vi "type_A_uncertainty.vi"(11 "X":dbl[](array[numeric]) format="%0.2f") -> (1 "u_A(x)":dbl, 3 "mean":dbl format="%0.2f")   [LabVIEW 2021]
uses:
  <vilib>/Analysis/NI_AALBase.lvlib
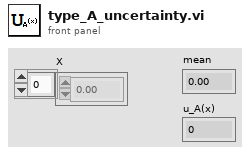
[diagram p1: front panel]
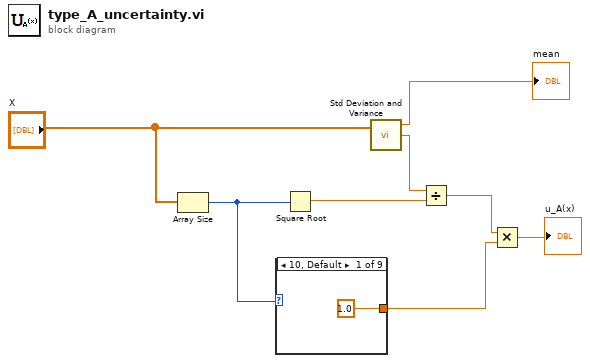
[diagram p0: block diagram]
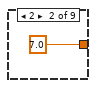
[diagram p2: hidden frame]
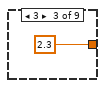
[diagram p3: hidden frame]
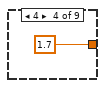
[diagram p4: hidden frame]
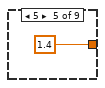
[diagram p5: hidden frame]
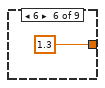
[diagram p6: hidden frame]
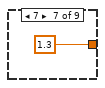
[diagram p7: hidden frame]
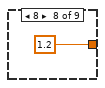
[diagram p8: hidden frame]
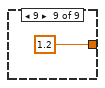
[diagram p9: hidden frame]
diagram:
  n1 = Array Size(array="X") -> (size(s)=w4:i32)
  n2 = case shown="10, Default" w4 {
    tunnel: [1.0 ("t") 7.0 ("t") 2.3 ("t") 1.7 ("t") 1.4 ("t") 1.3 ("t") 1.3 ("t") 1.2 ("t") 1.2 ("t")] -> w2
    frame 10, Default {
    }
    frame 2 {
    }
    frame 3 {
    }
    frame 4 {
    }
    frame 5 {
    }
    frame 6 {
    }
    frame 7 {
    }
    frame 8 {
    }
    frame 9 {
    }
  }
  n3 = Square Root(x=w4) -> (sqrt(x)=w6:dbl)
  n4 = call <vilib>:"Std Deviation and Variance.vi"("X"="X") -> ("mean"=→"mean":dbl, "standard deviation"=w7:dbl)  [unwired: 1 in, 1 out]
  n5 = Divide(x=w7, y=w6) -> (x/y=w5:dbl)
  n6 = Multiply(x=w5, y=w2) -> (x*y=→"u_A(x)":dbl)
